vi "Measure-laser-response.vi"(7 "LaserResponse in":refnum<class "HC-LaserResponse.lvclass">, 8 "error in (no error)":errorcluster, 9 "Device index":i32, 10 "File path":path, 11 "SM1000-control in":T1) -> (0 "error out":errorcluster, 3 "SM1000-control out":T1, 5 "LaserResponse":refnum<class "HC-LaserResponse.lvclass">)   [LabVIEW 2013, in "HardwareCharacterization.lvlib" / "HC-SM1000.lvclass"]
uses:
  HC-SM1000.lvclass
  Object-reference.ctl
  LaserPulseAnalyser/HC-LaserResponse.lvclass
  <vilib>/DAQmx/read.llb/DAQmx Read (Digital 1D U32 1Chan NSamp).vi
  <vilib>/DAQmx/read.llb/DAQmx Read (Analog 1D DBL 1Chan NSamp).vi
  <vilib>/DAQmx/miscellaneous.llb/DAQmx Fill In Error Info.vi
panel:
  out "Data points":i32
  out "Graph":dbl[](graph)
  out "Results saved":bool
  in  "Start job":bool
  out "Job busy":bool
  in  "Stop":bool
  out "Elapsed time":dbl caption="Elapsed time [ms]" format="%.2f"
  out "Initialized":bool
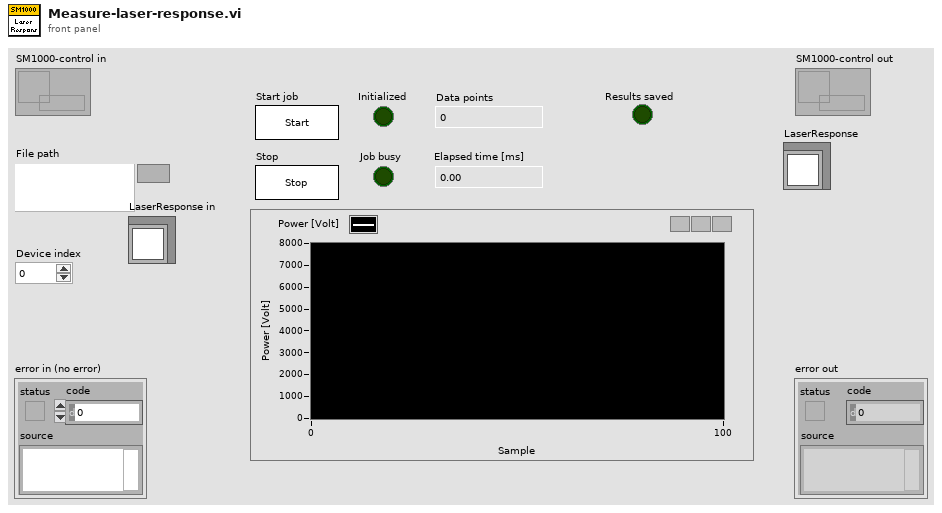
[diagram p1: front panel]
types:
  T1 = typedef "HardwareCharacterization.lvlib/HC-SM1000.lvclass/Object-reference.ctl" = refnum<data-value>
  T2 = enum8{"Enabled", "Disabled", "Disabled and Grayed Out"}
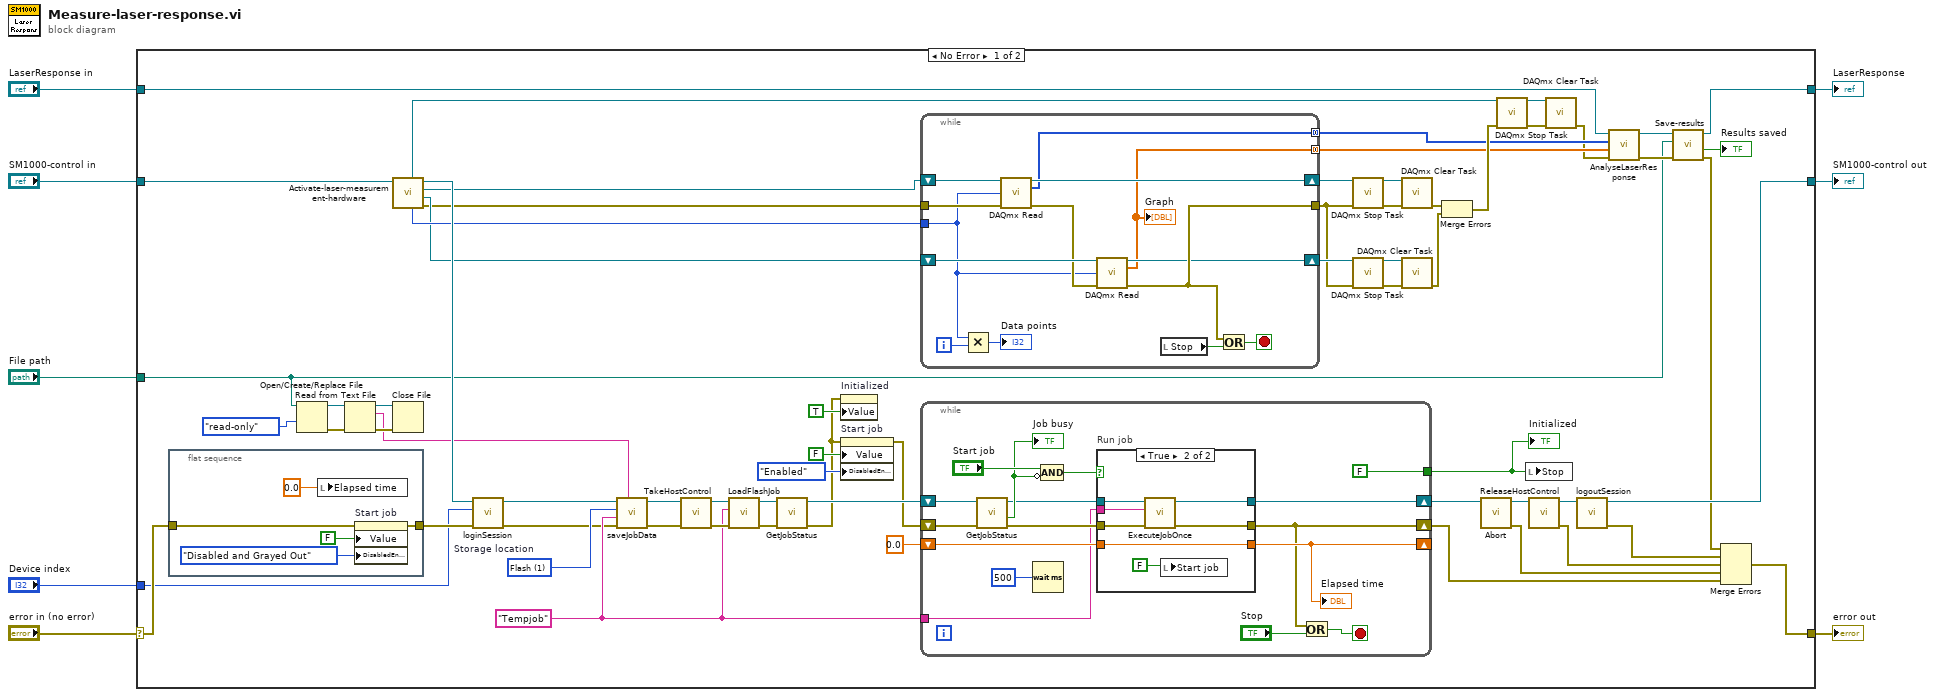
[diagram p0: block diagram]
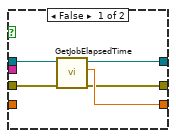
[diagram p2: hidden frame]
diagram:
  n1 = case shown="No Error" "error in (no error)" {
    selector: "error in (no error)" -> [w51 w123]
    tunnel: [w62 w123] -> w7
    tunnel: [w60 w122] -> w5
    tunnel: "SM1000-control in" -> [w47 w122]
    tunnel: "File path" -> [w13 _]
    tunnel: "Device index" -> [w50 _]
    tunnel: "LaserResponse in" -> [w22 w121]
    tunnel: [w17 w121] -> w1
    frame No Error {
      w69 = u16 1 items=["Flash"=1, "USB"=2]  # Storage location
      w66 = "Tempjob"
      n2 = flat-sequence {
        tunnel: [w90] -> w52
        tunnel: w51 -> [w89]
        frame #0 {
          n3 = local write "Elapsed time"(0.0 ("Elapsed time")) -> ()
          n4 = property on="Start job" class="Bool (strict)"(error in=w89, "Value"=FALSE, "DisabledEnum"=T2."Disabled and Grayed Out" ("Disabled")) -> (error out=w90:errorcluster)  [unwired: 1 in, 1 out]
        }
      }
      n5 = Open/Create/Replace File(file path (use dialog)=w13, access (0:read/write)=enum16{"read/write", "read-only", "write-only"}."read-only") -> (refnum out=w9:refnum<file>, error out=w15:errorcluster)  [unwired: 4 in, 1 out]
      n6 = Read from Text File(file (use dialog)=w9, error in=w15) -> (refnum out=w10:refnum<file>, text=w12:string, error out=w16:errorcluster)  [unwired: 2 in, 1 out]
      n7 = call "Activate-laser-measurement-hardware.vi"("SM1000-control in"=w47) -> ("error out"=w33:errorcluster, "Power"=w34:refnum<k21>, "Control"=w35:refnum<k21>, "SM1000-control out"=w46:T1, "Batch size"=w42:i32, "Timing"=w36:refnum<k21>)  [unwired: 5 in]
      n8 = Close File(refnum=w10, error in=w16) -> ()  [unwired: 2 out]
      n9 = call "loginSession.vi"("error in (no error)"=w52, "Device index"=w50, "SM1000-control in"=w46) -> ("error out"=w11:errorcluster, "SM1000-control out"=w57:T1)  [unwired: 7 in]
      n10 = call "saveJobData.vi"("Job data xml"=w12, "error in (no error)"=w11, "File name wo extension"=w66, "Storage location"=w69, "SM1000-control in"=w57) -> ("error out"=w44:errorcluster, "SM1000-control out"=w45:T1)  [unwired: 5 in]
      n11 = call "TakeHostControl.vi"("error in (no error)"=w44, "SM1000-control in"=w45) -> ("error out"=w71:errorcluster, "SM1000-control out"=w70:T1)  [unwired: 8 in]
      n12 = call "LoadFlashJob.vi"("error in (no error)"=w71, "Job name wo extension"=w66, "SM1000-control in"=w70) -> ("error out"=w73:errorcluster, "SM1000-control out"=w72:T1)  [unwired: 7 in]
      n13 = call "GetJobStatus.vi"("error in (no error)"=w73, "SM1000-control in"=w72) -> ("error out"=w48:errorcluster, "SM1000-control out"=w68:T1)  [unwired: 7 in, 1 out]
      n14 = property on="Initialized" class="Bool (strict)"(error in=w48, "Value"=TRUE ("Initialized")) -> ()  [unwired: 1 in, 2 out]
      n15 = property on="Start job" class="Bool (strict)"(error in=w48, "Value"=FALSE, "DisabledEnum"=T2."Enabled" ("Disabled")) -> (error out=w56:errorcluster)  [unwired: 1 in, 1 out]
      n16 = while {
        tunnel: w42 -> [w74]
        shift-right: [w85] -> w39
        shift-left: w35 -> [w87]
        shift-right: [w79] -> w31
        shift-left: w34 -> [w82]
        tunnel: [w77] -> w24 mode=concatenating
        tunnel: [w78] -> w25 mode=concatenating
        tunnel: w33 -> [w86]
        tunnel: [w80] -> w30
        i -> [w76]
        stop <- w84 stop-if-true
        n17 = Multiply(x=w74, y=w76) -> (x*y=→"Data points":i32)
        n18 = call-poly <vilib>:"DAQmx Read.vi"("task/channels in"=w87, "number of samples per channel"=w74, "error in"=w86) -> ("task out"=w85:refnum<k21>, "data"=w78:u32[], "error out"=w81:errorcluster)  [unwired: 10 in]
        n19 = call-poly <vilib>:"DAQmx Read.vi"("task/channels in"=w82, "number of samples per channel"=w74, "error in"=w81) -> ("task out"=w79:refnum<k21>, "data"=w77:dbl[], "error out"=w80:errorcluster)  [unwired: 10 in]
        "Graph" <- w77
        n20 = local read "Stop"() -> (w83:bool)
        n21 = Or(x=w80, y=w83) -> (x .or. y?=w84:bool)
      }
      n22 = while {
        shift-right: [w93] -> w43
        shift-left: w56 -> [w107]
        shift-right: [w94] -> w58
        shift-left: w68 -> [w108]
        shift-right: [w98] -> _
        shift-left: 0.0 ("Elapsed time") -> [w99]
        tunnel: w66 -> [w97]
        tunnel: [FALSE] -> w54
        stop <- w102 stop-if-true
        n23 = call "GetJobStatus.vi"("error in (no error)"=w107, "SM1000-control in"=w108) -> ("error out"=w101:errorcluster, "Busy?"=w104:bool, "SM1000-control out"=w100:T1)  [unwired: 7 in]
        "Job busy" <- w104
        n24 = Wait (ms)(milliseconds to wait=u32 500) -> ()  [unwired: 1 out]
        n25 = Compound Arithmetic op=AND("Start job", invert w104) -> (w105:bool)
        n26 = case "Run job" shown="True" w105 {
          tunnel: w101 -> [w111 w117]
          tunnel: [w109 w116] -> w93
          tunnel: [w110 w115] -> w94
          tunnel: w100 -> [w113 w118]
          tunnel: [w112 w120] -> w98
          tunnel: w99 -> [_ w120]
          tunnel: w97 -> [_ w119]
          frame False {
            n27 = call "GetJobElapsedTime.vi"("error in (no error)"=w111, "SM1000-control in"=w113) -> ("error out"=w109:errorcluster, "Elapsed time"=w112:dbl, "SM1000-control out"=w110:T1)  [unwired: 7 in]
          }
          frame True {
            n28 = call "ExecuteJobOnce.vi"("error in (no error)"=w117, "Job name wo extension"=w119, "SM1000-control in"=w118) -> ("error out"=w116:errorcluster, "SM1000-control out"=w115:T1)  [unwired: 7 in]
            n29 = local write "Start job"(FALSE) -> ()
          }
        }
        "Elapsed time" <- w98
        n30 = Or(x=w93, y="Stop") -> (x .or. y?=w102:bool)
      }
      "Initialized" <- w54
      n31 = call <vilib>:"DAQmx Stop Task.vi"("task/channels in"=w39, "error in"=w30) -> ("task out"=w38:refnum<k21>, "error out"=w37:errorcluster)  [unwired: 12 in]
      n32 = call <vilib>:"DAQmx Stop Task.vi"("task/channels in"=w31, "error in"=w30) -> ("task out"=w29:refnum<k21>, "error out"=w32:errorcluster)  [unwired: 12 in]
      n33 = call <vilib>:"DAQmx Clear Task.vi"("task in"=w38, "error in"=w37) -> ("error out"=w28:errorcluster)  [unwired: 13 in]
      n34 = call <vilib>:"DAQmx Clear Task.vi"("task in"=w29, "error in"=w32) -> ("error out"=w27:errorcluster)  [unwired: 13 in]
      n35 = Merge Errors(w28, w27) -> (w26:errorcluster)
      n36 = call "Abort.vi"("SM1000-control in"=w58) -> ("error out"=w63:errorcluster, "SM1000-control out"=w65:T1)  [unwired: 9 in]
      n37 = call <vilib>:"DAQmx Stop Task.vi"("task/channels in"=w36, "error in"=w26) -> ("task out"=w40:refnum<k21>, "error out"=w41:errorcluster)  [unwired: 12 in]
      n38 = local write "Stop"(w54) -> ()
      n39 = call "ReleaseHostControl.vi"("SM1000-control in"=w65) -> ("error out"=w64:errorcluster, "SM1000-control out"=w61:T1)  [unwired: 9 in]
      n40 = call <vilib>:"DAQmx Clear Task.vi"("task in"=w40, "error in"=w41) -> ("error out"=w23:errorcluster)  [unwired: 13 in]
      n41 = call "logoutSession.vi"("SM1000-control in"=w61) -> ("error out"=w59:errorcluster, "SM1000-control out"=w60:T1)  [unwired: 9 in]
      n42 = call "AnalyseLaserResponse.vi"("error in (no error)"=w23, "Power"=w24, "Constrol"=w25, "HC-LaserPulse in"=w22) -> ("error out"=w20:errorcluster, "HC-LaserPulse out"=w21:refnum<class "HC-LaserResponse.lvclass">)  [unwired: 5 in, 1 out]
      n43 = call "Save-results.vi"("error in (no error)"=w20, "Base file path"=w13, "LaserResponse in"=w21) -> ("error out"=w19:errorcluster, "Valid?"=→"Results saved":bool, "LaserResponse"=w17:refnum<class "HC-LaserResponse.lvclass">)  [unwired: 6 in]
      n44 = Merge Errors(w19, w59, w64, w63, w43) -> (w62:errorcluster)
    }
    frame Error {
    }
  }
  "error out" <- w7
  "SM1000-control out" <- w5
  "LaserResponse" <- w1
